vi "Statistical Analysis.vi"(7 "error in (no error)":errorcluster, 10 "Graph Data In":T1) -> (0 "error out":errorcluster, 3 "Graph Data Out":T1)   [LabVIEW 2018]
doc: "Computes basic statistics (mean, RMS, min, max, peak to peak and frequency) for each waveform in the input data and outputs annotations."
uses:
  controls/Graph Data.ctl
  <vilib>/Utility/miscctls.llb/LVAnnotationListTypeDef.ctl
  <vilib>/Utility/miscctls.llb/LVCursorListTypeDef.ctl
panel:
  # "(Scroll up to see large data in/out clusters)"
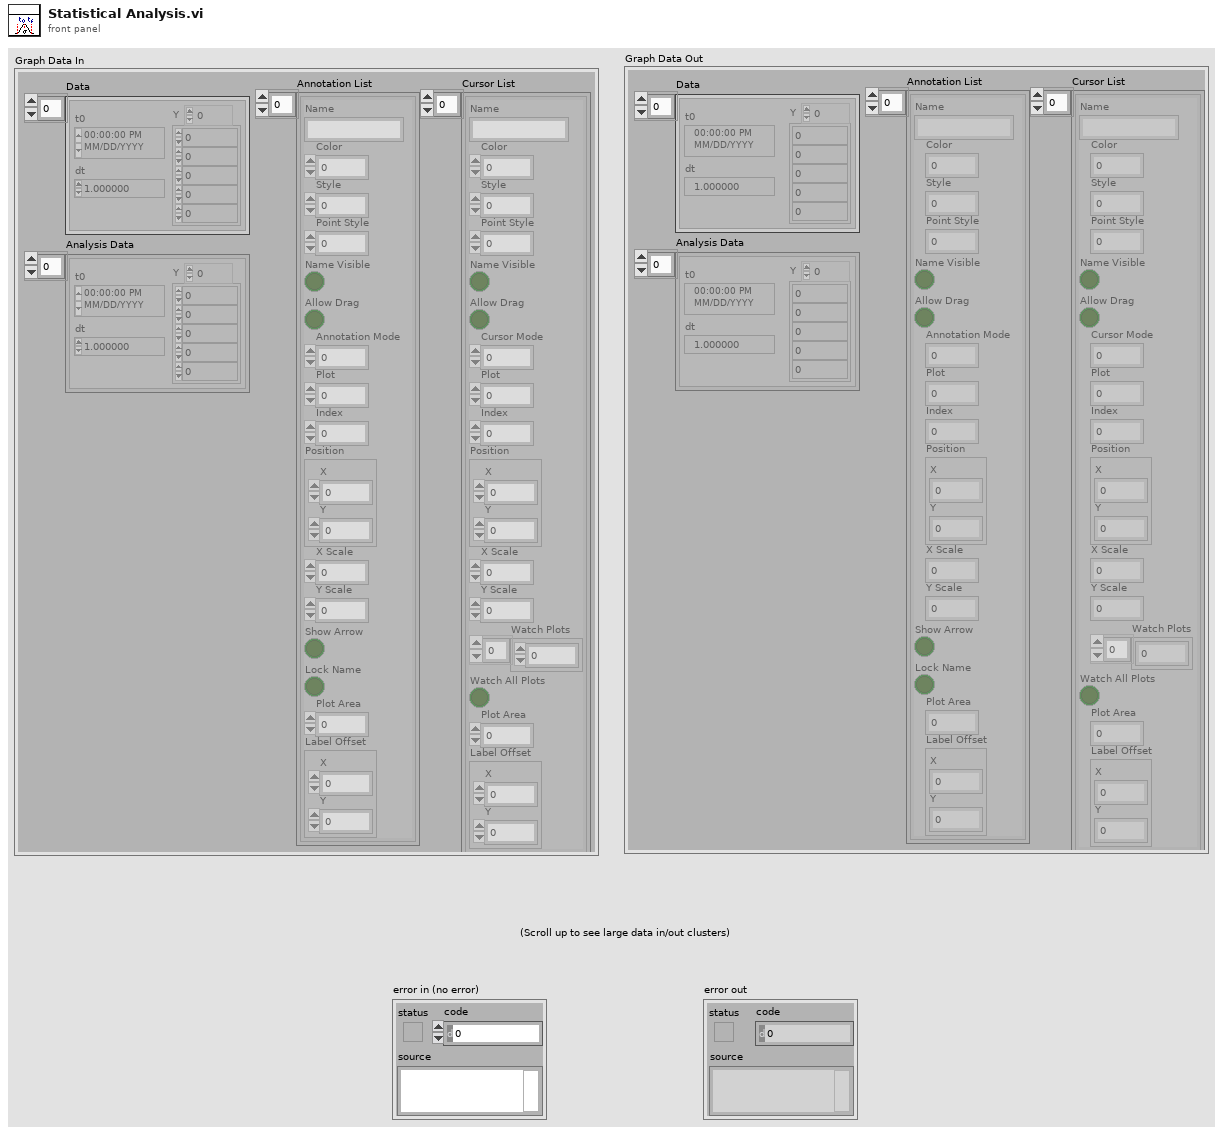
[diagram p1: front panel]
types:
  T1 = typedef "Graph Data.ctl" = cluster{"Data":waveform(dbl)[], "Annotation List":T2, "Cursor List":T3, "Analysis Data":waveform(dbl)[]}
  T2 = typedef "LVAnnotationListTypeDef.ctl" = cluster{"Name":string, "Color":u32, "Style":u8, "Point Style":u8, "Name Visible":bool, "Allow Drag":bool, "Annotation Mode":u32, "Plot":i32, "Index":i32, "Position":cluster{"X":dbl, "Y":dbl}, "X Scale":u32, "Y Scale":u32, "Show Arrow":bool, "Lock Name":bool, "Plot Area":i32, "Label Offset":cluster{"X":dbl, "Y":dbl}}[]
  T3 = typedef "LVCursorListTypeDef.ctl" = cluster{"Name":string, "Color":u32, "Style":u8, "Point Style":u8, "Name Visible":bool, "Allow Drag":bool, "Cursor Mode":u32, "Plot":i32, "Index":i32, "Position":cluster{"X":dbl, "Y":dbl}, "X Scale":u32, "Y Scale":u32, "Watch Plots":i32[], "Watch All Plots":bool, "Plot Area":i32, "Label Offset":cluster{"X":dbl, "Y":dbl}}[]
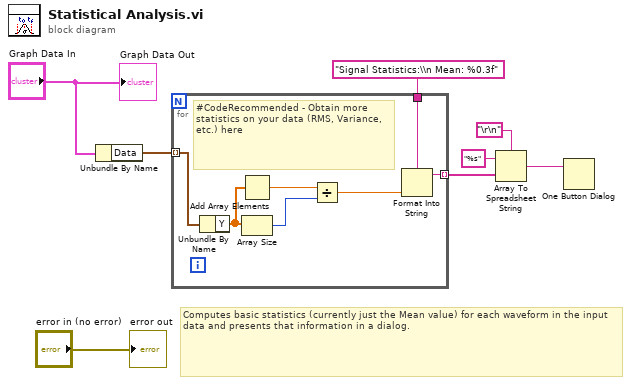
[diagram p0: block diagram]
diagram:
  # "Computes basic statistics (currently just the Mean value) for each waveform in the input data and presents that information in a dialog."
  n1 = Unbundle By Name("Graph Data In") -> ("Data"=w8:waveform(dbl)[])
  n2 = for {
    tunnel: w8 -> [w13] mode=indexing
    tunnel: "Signal Statistics:\\n Mean: %0.3f" ("Signal Statistics") -> [w15]
    tunnel: [w14] -> w4 mode=indexing
    # "#CodeRecommended - Obtain more statistics on your data (RMS, Variance, etc.) here"
    n3 = Unbundle By Name(w13) -> ("Y"=w9:dbl[])
    n4 = Add Array Elements(numeric array=w9) -> (sum=w12:dbl)
    n5 = Array Size(array=w9) -> (size(s)=w10:i32)
    n6 = Divide(x=w12, y=w10) -> (x/y=w11:dbl)
    n7 = Format Into String(format string=w15, w11) -> (resulting string=w14:string)  [unwired: 2 in, 1 out]
  }
  n8 = Array To Spreadsheet String(delimiter (Tab)="\r\n", array=w4, 3:"%s" ("format string")) -> (spreadsheet string=w1:string)
  n9 = One Button Dialog(message=w1) -> ()  [unwired: 1 in, 1 out]
  "error out" <- "error in (no error)"
  "Graph Data Out" <- "Graph Data In"
